vi "GenCM-Save config.vi"(0 "configuration file path":path=path "C:/PXI Connections.txt", 5 "Analog Connections":cluster{"Outputs":string[], "Inputs":string[]}[](array[cluster]), 7 "Endpoints":cluster{"Inputs":string[], "Outputs":string[]}, 11 "error in (no error)":errorcluster) -> (15 "error out":errorcluster)   [LabVIEW 2020]
uses:
  <vilib>/Utility/config.llb/Write Key (I32).vi
  <vilib>/Utility/config.llb/NI_LVConfig.lvlib
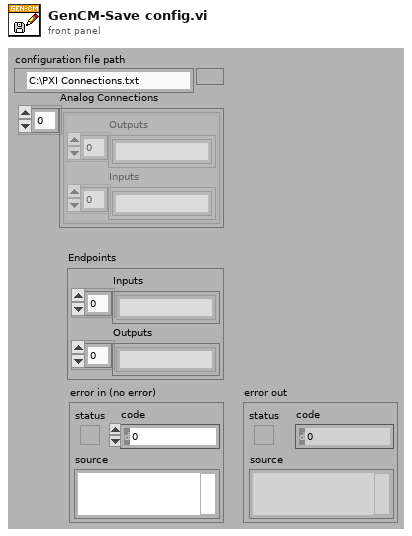
[diagram p1: front panel]
types:
  T1 = typedef "NI_LVConfig.lvlib/Config Data RefNum.ctl" = refnum<k1>
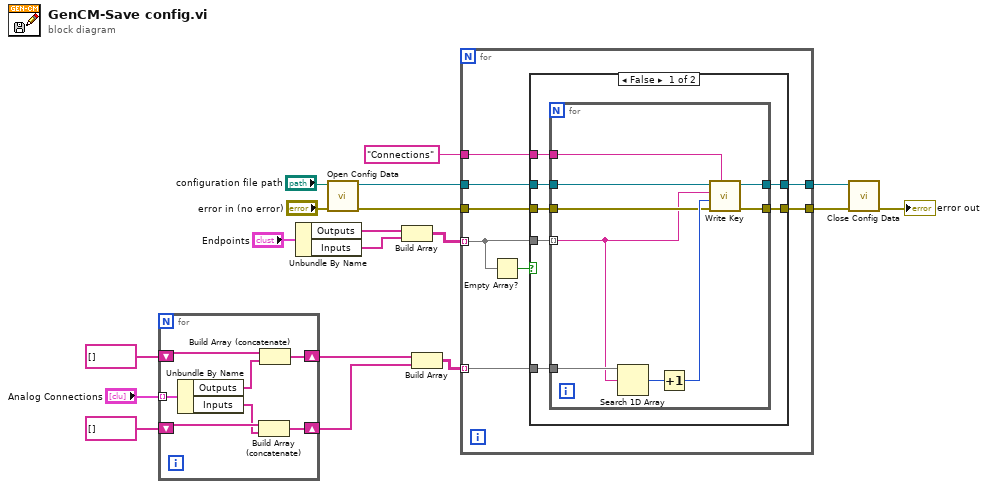
[diagram p0: block diagram]
diagram:
  n1 = for {
    tunnel: "Analog Connections" -> [w25] mode=indexing
    shift-right: [w23] -> w4
    shift-left: string[] [] -> [w22]
    shift-right: [w21] -> w3
    shift-left: string[] [] -> [w20]
    n2 = Unbundle By Name(w25) -> ("Outputs"=w24:string[], "Inputs"=w19:string[])
    n3 = Build Array (concatenate)(w20, w19) -> (w21:string[])
    n4 = Build Array (concatenate)(w22, w24) -> (w23:string[])
  }
  n5 = Unbundle By Name("Endpoints") -> ("Outputs"=w9:string[], "Inputs"=w8:string[])
  n6 = call <vilib>:"Open Config Data.vi"("error in (no error)"="error in (no error)", "configuration file path"="configuration file path") -> ("error out"=w6:errorcluster, "refnum"=w7:T1)  [unwired: 7 in, 1 out]
  n7 = Build Array(w9, w8) -> (w5:string[][])
  n8 = Build Array(w4, w3) -> (w2:string[][])
  n9 = for {
    tunnel: [w33] -> w12
    tunnel: [w32] -> w11
    tunnel: w7 -> [w27]
    tunnel: w6 -> [w26]
    tunnel: w5 -> [w30] mode=indexing
    tunnel: w2 -> [w29] mode=indexing
    tunnel: "Connections" ("section") -> [w28]
    n10 = Empty Array?(array=w30) -> (empty?=w31:bool)
    n11 = case shown="False" w31 {
      tunnel: w29 -> [w40 _]
      tunnel: w27 -> [w39 w51]
      tunnel: w26 -> [w38 w50]
      tunnel: w30 -> [w37 _]
      tunnel: [w36 w51] -> w33
      tunnel: [w35 w50] -> w32
      tunnel: w28 -> [w34 _]
      frame False {
        n12 = for {
          tunnel: w37 -> [w42] mode=indexing
          tunnel: w40 -> [w48]
          tunnel: w39 -> [w47]
          tunnel: [w44] -> w36
          tunnel: w38 -> [w45]
          tunnel: [w43] -> w35
          tunnel: w34 -> [w41]
          n13 = Search 1D Array(1D array=w48, element=w42) -> (index of element=w49:i32)  [unwired: 1 in]
          n14 = Increment(x=w49) -> (x+1=w46:i32)
          n15 = call-poly <vilib>:"Write Key.vi"("section"=w41, "error in (no error)"=w45, "value"=w46, "key"=w42, "refnum"=w47) -> ("error out"=w43:errorcluster, "refnum out"=w44:T1)  [unwired: 4 in, 1 out]
        }
      }
      frame True {
      }
    }
  }
  n16 = call <vilib>:"Close Config Data.vi"("error in (no error)"=w11, "refnum"=w12) -> ("error out"=→"error out":errorcluster)  [unwired: 8 in, 1 out]
